vi "_script_update_api_doc.vi"() -> ()   [LabVIEW 2014]
uses:
  JKI State Machine++.lvlib
panel:
  out "States":string
  out "appended array":path[](array[path])
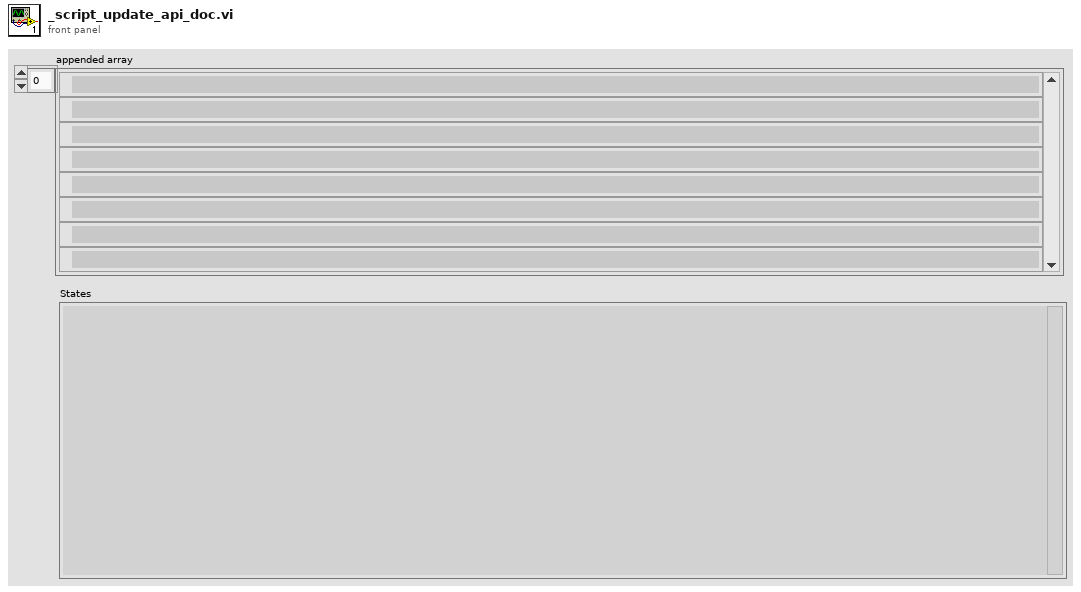
[diagram p1: front panel]
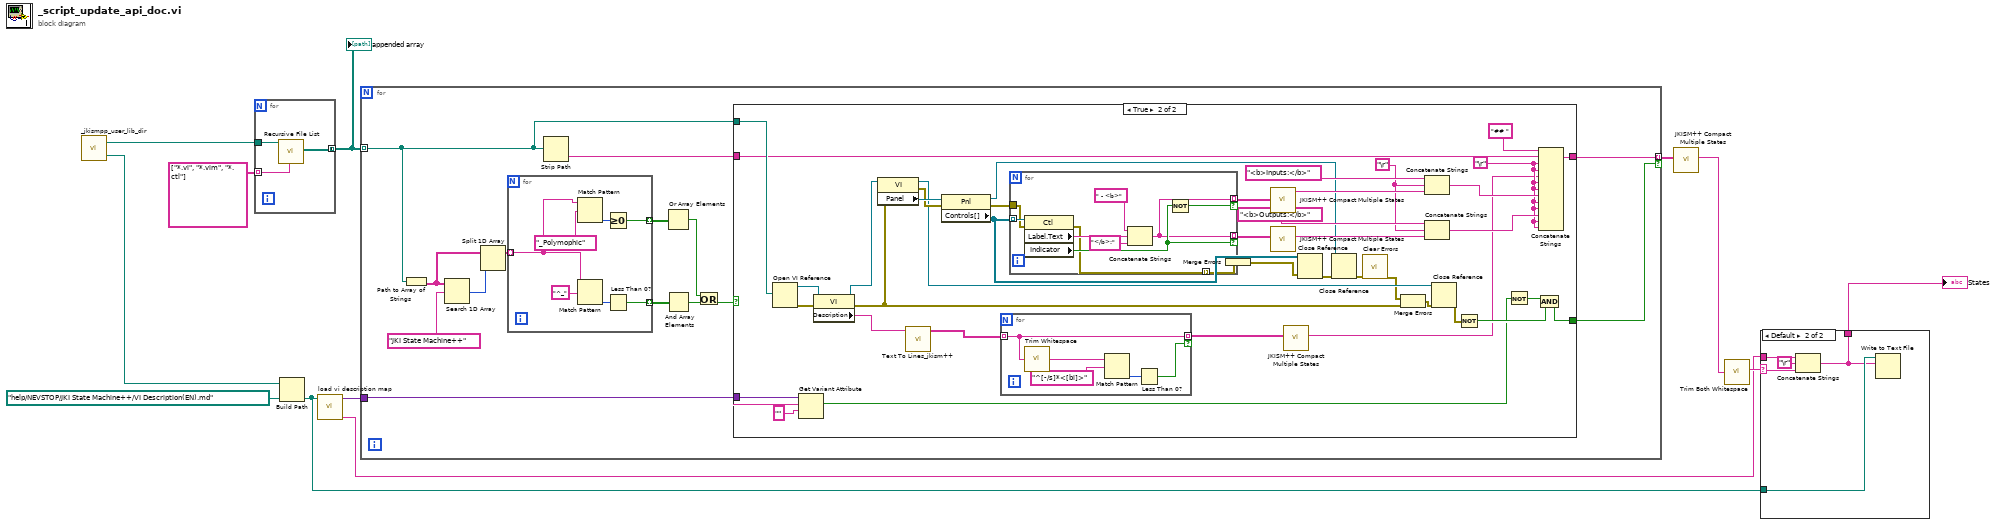
[diagram p0: block diagram]
diagram:
  n1 = call "_jkismpp_user_lib_dir.vi"() -> ("<LabVIEW>"=w2:path, "jkismpp_user.lib_dir"=w1:path)  [unwired: 2 in]
  n2 = for {
    tunnel: w1 -> [w15]
    tunnel: string[] ["*.vi", "*.vim", "*.ctl"] -> [w14] mode=indexing
    tunnel: [w13] -> w11 mode=concatenating
    n3 = call <vilib>:"Recursive File List.vi"("pattern"=w14, "Folder Path"=w15) -> ("All Files in Dir"=w13:path[])  [unwired: 5 in, 4 out]
  }
  "appended array" <- w11
  n4 = Build Path(base path=w2, name or relative path=path "help/NEVSTOP/JKI State Machine++/VI Description(EN).md" ("Path")) -> (appended path=w6:path)
  n5 = call "load vi description map.vi"("Path"=w6) -> ("text"=w4:string, "variant"=w8:variant)  [unwired: 9 in]
  n6 = for {
    tunnel: w11 -> [w27] mode=indexing
    tunnel: [w29] -> w9 mode=indexing if=w20
    tunnel: w8 -> [w19]
    n7 = Path to Array of Strings(0:w27) -> (2:w24:string[])  [unwired: 1 out]
    n8 = Search 1D Array(1D array=w24, element="JKI State Machine++") -> (index of element=w25:i32)  [unwired: 1 in]
    n9 = Split 1D Array(array=w24, index=w25) -> (second subarray=w23:string[])  [unwired: 1 out]
    n10 = for {
      tunnel: [w34] -> w28 mode=indexing
      tunnel: w23 -> [w31] mode=indexing
      tunnel: [w30] -> w18 mode=indexing
      n11 = Match Pattern(string=w31, regular expression="_Polymophic") -> (offset past match=w33:i32)  [unwired: 1 in, 3 out]
      n12 = Match Pattern(string=w31, regular expression="^_") -> (offset past match=w35:i32)  [unwired: 1 in, 3 out]
      n13 = Greater Or Equal To 0?(x=w33) -> (x >= 0?=w30:bool)
      n14 = Less Than 0?(x=w35) -> (x < 0?=w34:bool)
    }
    n15 = Strip Path(path=w27) -> (name=w21:string)  [unwired: 1 out]
    n16 = Or Array Elements(Boolean array=w18) -> (logical OR=w16:bool)
    n17 = And Array Elements(Boolean array=w28) -> (logical AND=w22:bool)
    n18 = Or(x=w16, y=w22) -> (x .or. y?=w17:bool)
    n19 = case shown="True" w17 {
      tunnel: [_ w76] -> w29
      tunnel: w27 -> [_ w75]
      tunnel: [_ w66] -> w20
      tunnel: w21 -> [_ w69]
      tunnel: w19 -> [_ w70]
      frame False {
      }
      frame True {
        w45 = "\r"
        w44 = "\r"
        n20 = Open VI Reference(vi path=w75) -> (vi reference=w73:refnum<vi>, error out=w74:errorcluster)  [unwired: 5 in]
        n21 = Get Variant Attribute(Variant=w70, name=w69, default value (empty Variant)="" ("string")) -> (found=w63:bool)  [unwired: 1 in, 3 out]
        n22 = property class="VI"(reference=w73, error in=w74) -> (reference out=w65:refnum<vi>, error out=w40:errorcluster, "Description"=w67:string)
        n23 = property class="VI"(reference=w65, error in=w40) -> (reference out=w46:refnum<vi>, error out=w53:errorcluster, "Panel"=w64:refnum<vi>)
        n24 = call "Text To Lines_jkism++.vi"("string"=w67) -> ("Lines"=w43:string[])  [unwired: 9 in, 1 out]
        n25 = property class="Pnl"(reference=w64, error in=w53) -> (reference out=w47:refnum<vi>, error out=w50:errorcluster, "Controls[]"=w52:refnum<vi>[])
        n26 = for {
          tunnel: w43 -> [w82] mode=indexing
          tunnel: [w82] -> w42 mode=indexing if=w78
          n27 = call <vilib>:"Trim Whitespace.vi"("string"=w82) -> ("trimmed string"=w81:string)  [unwired: 1 in]
          n28 = Match Pattern(string=w81, regular expression="^[-/s]*<[bi]>") -> (offset past match=w79:i32)  [unwired: 1 in, 3 out]
          n29 = Less Than 0?(x=w79) -> (x < 0?=w78:bool)
        }
        n30 = for {
          tunnel: w52 -> [w91] mode=indexing
          tunnel: [w87] -> w61 mode=indexing if=w88
          tunnel: [w87] -> w60 mode=indexing if=w89
          tunnel: w50 -> [w85]
          tunnel: [w84] -> w49 mode=indexing
          n31 = property class="Ctl"(reference=w91, error in=w85) -> (error out=w84:errorcluster, "Label.Text"=w90:string, "Indicator"=w89:bool)  [unwired: 1 out]
          n32 = Concatenate Strings(" - <b>" ("string"), w90, "</b>:" ("string")) -> (w87:string)
          n33 = Not(x=w89) -> (.not. x?=w88:bool)
        }
        n34 = Merge Errors(w49) -> (w48:errorcluster)
        n35 = call "JKISM++ Compact Multiple States.vi"("States in Lines"=w61) -> ("States"=w58:string)  [unwired: 9 in]
        n36 = call "JKISM++ Compact Multiple States.vi"("States in Lines"=w60) -> ("States"=w59:string)  [unwired: 9 in]
        n37 = call "JKISM++ Compact Multiple States.vi"("States in Lines"=w42) -> ("States"=w41:string)  [unwired: 9 in]
        n38 = Close Reference(reference=w52, error in (no error)=w48) -> (error out=w51:errorcluster)
        n39 = Close Reference(reference=w47, error in (no error)=w51) -> (error out=w39:errorcluster)
        n40 = call <vilib>:"Clear Errors.vi"("error in (no error)"=w39) -> ("error out"=w37:errorcluster)  [unwired: 5 in, 1 out]
        n41 = Merge Errors(w37, w40) -> (w38:errorcluster)
        n42 = Concatenate Strings("<b>Inputs:</b>" ("string"), w45, w58) -> (w55:string)
        n43 = Concatenate Strings("<b>Outputs:</b>" ("string"), w45, w59) -> (w54:string)
        n44 = Close Reference(reference=w46, error in (no error)=w38) -> (error out=w72:errorcluster)
        n45 = Not(x=w72) -> (.not. x?=w71:bool)
        n46 = Not(x=w63) -> (.not. x?=w62:bool)
        n47 = And(x=w62, y=w71) -> (x .and. y?=w66:bool)
        n48 = Concatenate Strings("## " ("string"), w69, w44, w44, w41, w44, w44, w55, w44, w44, w54, w44, w44) -> (w76:string)
      }
    }
  }
  n49 = call "JKISM++ Compact Multiple States.vi"("States in Lines"=w9) -> ("States"=w7:string)  [unwired: 9 in]
  n50 = call "Trim Both Whitespace.vi"("string"=w7) -> ("trimmed string"=w5:string)  [unwired: 1 in]
  n51 = case shown="Default" w5 {
    selector: w5 -> [_ w95]
    tunnel: w6 -> [_ w96]
    tunnel: w4 -> [w92 w94]
    tunnel: [w92 w93] -> w3
    frame "" {
    }
    frame Default {
      n52 = Concatenate Strings(w94, "\r", w95) -> (w93:string)
      n53 = Write to Text File(file (use dialog)=w96, text=w93) -> ()  [unwired: 2 in, 3 out]
    }
  }
  "States" <- w3
